vi "LV to ITX 2D AutoPlot.vi"(4 "Notes":string, 6 "X,Y,Z Labels":string[](array[string])=["x", "y"], 8 "error in":errorcluster, 10 "2D, X, Y (Cluster)":T1={"2D Array"=[], "X 1D Array"=[0.0, 1.0], "Y 1D Array"=[0.0, 1.0]}, 11 "path":path) -> (0 "error out":errorcluster, 3 "file":path)   [LabVIEW 2016, in "Data.ITX.lvclass"]
doc: "Write your 2D data to ITX file. This AutoPlot VI adds commands that will automatically create in Igor an intensity graph with X and Y axes scaled by the 1D arrays, allowing you to quickly view your data.\n\n-- path: base path to save data\n-- filename: base filename\n-- Notes: add any notes here to help you remember what experiment you did\n-- 2D Array: Intensity data\n-- X,Y Arrays: These are used to apply an appropriate scaling to the intensity graph\n-- X,Y wavenames: Default \"x_\" and \"y_\" are fine.\n-- X,Y,Z Labels: Labels for plotting in Igor."
uses:
  Data.ITX.lvclass
  Data/Data.lvclass
  Data/Typedefs/File Type--enum.ctl
panel:
  in  "input command string":string="Display;AppendImage '#wave2D#'\nModifyGraph width=216,height={Aspect,1}\nLabel bottom \"#labelX#\"\nLabel left \"#labelY#\"\nModifyImage '#wave2D#' ctab= {*,*,Rainbow,1}\nModifyGraph mirror=1"
  # "Below are relevant for creating graphs in Igor"
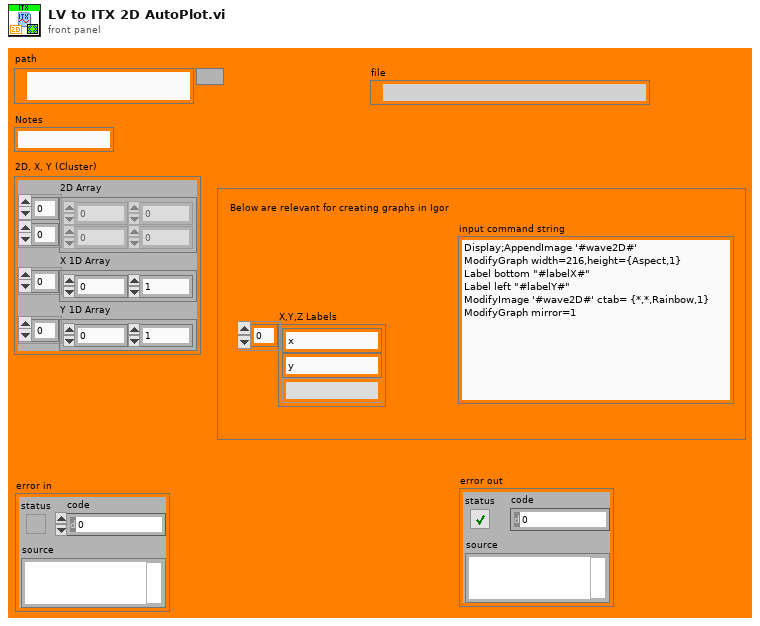
[diagram p1: front panel]
types:
  T1 = cluster{"2D Array":dbl[][], "X 1D Array":dbl[], "Y 1D Array":dbl[]}
  T2 = typedef "Data.lvclass/File Type--enum.ctl" = enum16{"DAT", "ITX", "HDF5", "TDMS", "VI", "PGSQL"}
  T3 = cluster{void, "X wavename":string, "X  Array name":string}
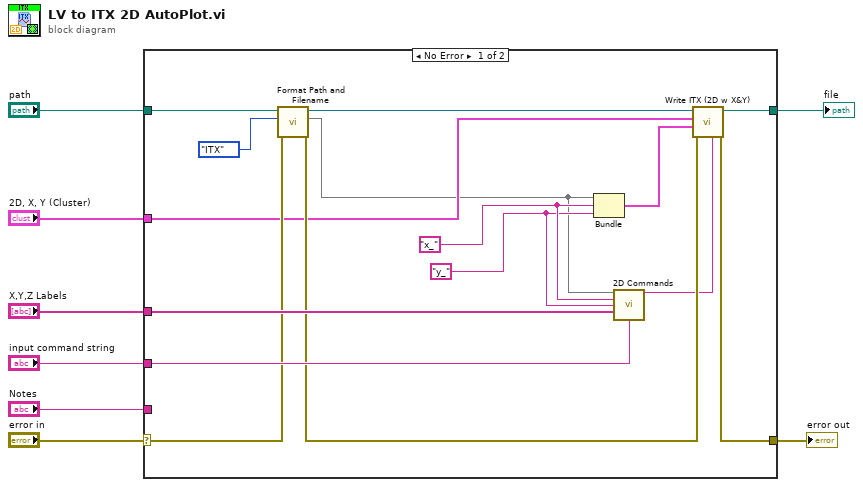
[diagram p0: block diagram]
diagram:
  n1 = case shown="No Error" "error in" {
    selector: "error in" -> [w20 w25]
    tunnel: "path" -> [w23 w24]
    tunnel: "Notes" -> [_ _]
    tunnel: "X,Y,Z Labels" -> [w22 _]
    tunnel: "input command string" -> [w21 _]
    tunnel: [w16 w25] -> w4
    tunnel: [w15 w24] -> w3
    tunnel: "2D, X, Y (Cluster)" -> [w13 _]
    frame No Error {
      w12 = "x_" ("X wavename")
      w11 = "y_" ("X  Array name")
      n2 = call "Format Path and Filename.vi"("error in"=w20, 10:File_Type--enum."ITX" ("Type"), "Data in"=w23) -> ("error out"=w17:errorcluster, 2:w9, "Data out"=w18:refnum<class "Data.lvclass">)  [unwired: 6 in]
      n3 = Bundle(w9, "X wavename"=w12, "X  Array name"=w11) -> (w10:T3)  [unwired: 1 in]
      n4 = call "2D Commands.vi"("2D wavename"=w9, "X wavename"=w12, "Y wavename"=w11, "X,Y,Z Labels"=w22, "input string"=w21) -> ("result string"=w14:string)  [unwired: 1 in, 9 out]
      n5 = call "Write ITX (2D w X&Y).vi"("Commands"=w14, "error in"=w17, "Wavenames"=w10, "2D, X, Y (Cluster)"=w13, "filename"=w18) -> ("error out"=w16:errorcluster, "file out"=w15:path)  [unwired: 4 in, 1 out]
    }
    frame Error {
    }
  }
  "file" <- w3
  "error out" <- w4
